vi "ProcessName.vi"() -> (1 "process name":string)   [LabVIEW 2017, in "DeviceHealth.lvlib"]
uses:
  <vilib>/addons/InsightCM/Devices/Shared/Common/DeviceHealth/DeviceHealth.lvlib
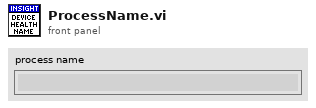
[diagram p1: front panel]
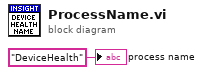
[diagram p0: block diagram]
diagram:
  "process name" <- "DeviceHealth" ("ProcessName")
